vi "Process Helper.vi"(8 "error in (no error)":errorcluster, 11 "Plugin in":refnum<class "Sequencer with Output Values.lvclass">) -> (0 "error out":errorcluster, 1 "Digital Values to Write":bool[](array[boolean]), 2 "Analog Values to Write":dbl[](array[numeric]), 3 "Plugin out":refnum<class "Sequencer with Output Values.lvclass">, 4 "New Flatterned Params (Empty if no change)":string)   [LabVIEW 2020, in "Sequencer with Output Values.lvlib" / "Sequencer with Output Values.lvclass"]
uses:
  Sequencer with Output Values.lvclass
  C:/Program Files/National Instruments/LabVIEW 2024/vi.lib/FlexLogger/SDK/PluginSDK.lvlibp/PEFClasses/SDK/Processing Element/Processing Element.lvclass
  Sequencer with Output Values.lvclass/Sequencer with Output Values.ctl
  <vilib>/FlexLogger/SDK/PluginSDK.lvlibp/PEFClasses/SDK/Processing Element/Read Alias.vi
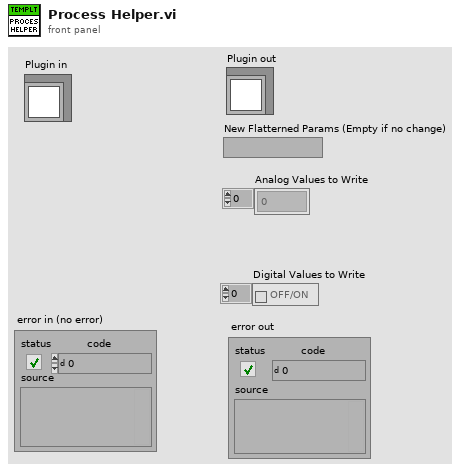
[diagram p1: front panel]
types:
  T1 = typedef "Sequencer with Output Values.lvlib/Sequencer with Output Values.lvclass/Cust UI.ctl" = refnum<vi>
  T2 = typedef "Sequencer with Output Values.lvlib/Sequencer with Output Values.lvclass/Params.ctl" = cluster{"Step Values":T3[], "Only Execute When Test Running":bool, "Reset Sequence When Test Starts":bool, "Current Sequence ID":u32, "Total Iterations":u32, "Current Step Start Timestamp":dbl, "Number of Sequence Steps":i32, "Num of Analog Channels":i32, "Num of Digital Channels":i32, "Delay Before Starting Sequence":dbl, "Show UI":bool, "Time Remaining":dbl, "Test Running":bool, "Pause Timestamp":dbl, "Default Analog Values":dbl[], "Default Digital Values":bool[]}
  T3 = typedef "Sequencer with Output Values.lvlib/Sequencer with Output Values.lvclass/Step Settings.ctl" = cluster{"Duration":dbl, "Mode":string, "Delay Between Values":dbl, "Analog Values":string[], "Digital Values":string[]}
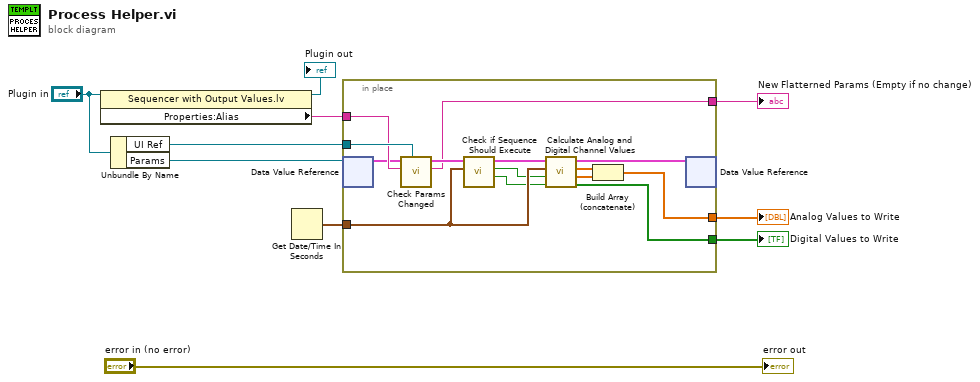
[diagram p0: block diagram]
diagram:
  n1 = property class="Sequencer with Output Values.lv"(reference="Plugin in") -> (reference out=→"Plugin out":refnum<class "Sequencer with Output Values.lvclass">, "Properties:Alias"=w7:string)  [unwired: 1 in, 1 out]
  n2 = Unbundle By Name("Plugin in") -> ("UI Ref"=w8:T1, "Params"=w9:refnum<data-value>)
  n3 = Get Date/Time In Seconds() -> (seconds since 1Jan1904=w4:timestamp)
  n4 = in-place {
    in-place-border: w8 -> [w24]
    in-place-border: w7 -> [w23]
    in-place-border: w4 -> [w18]
    in-place-border: [w21] -> w6
    in-place-border: [w20] -> w5
    in-place-border: [w13] -> w2
    n5 = in-place-dvr #1(w9) -> (w12:T2)  [unwired: 1 out]
    n6 = call "Check Params Changed.vi"("UI Ref"=w24, "Alias"=w23, "Settings in"=w12) -> ("New Flatterned Params (Empty if no change)"=w13:string, "Settings out"=w19:T2)  [unwired: 7 in]
    n7 = call "Check if Sequence Should Execute.vi"("Current time"=w18, "Settings in"=w19) -> ("Use Default Values"=w11:bool, "Execute Sequence"=w14:bool, "Settings out"=w17:T2)  [unwired: 7 in]
    n8 = call "Calculate Analog and Digital Channel Values.vi"("Use Default Values"=w11, "Execute Sequence"=w14, "current time"=w18, "Settings in"=w17) -> ("Digital Values to Write"=w20:bool[], "Analog Values to Write"=w15:dbl[], "Sequence State Channels to Write"=w16:dbl[], "Settings out"=w22:T2)  [unwired: 4 in]
    n9 = Build Array (concatenate)(w16, w15) -> (w21:dbl[])
    n10 = in-place-dvr #1(w22) -> ()  [unwired: 2 out]
  }
  "Digital Values to Write" <- w5
  "Analog Values to Write" <- w6
  "New Flatterned Params (Empty if no change)" <- w2
  "error out" <- "error in (no error)"
